vi "TEST SCREEN UPDATE_2.vi"(0 "Station in 1":refnum<class "Modbus Master.lvclass">, 3 "Staion  in error 2":errorcluster, 5 "Staion  in error 3":errorcluster, 6 "DataBase connection in":T11, 7 "Database error in":errorcluster, 21 "Staion  in error 1":errorcluster) -> (1 "Staion Error Out 1":errorcluster, 20 "Staion Out 1":refnum<k5>, 22 "Staion Out 2":refnum<k5>, 23 "Staion Error Out 2":errorcluster, 24 "Staion Out 3":refnum<k5>, 25 "Staion Error Out 3":errorcluster, 26 "Database connection out":T11, 27 "Database error out":errorcluster)   [LabVIEW 2024]
uses:
  <vilib>/addons/database/Connection.llb/Conn ObjectReference.ctl
  Controls/OP10_Cluster.ctl
  Controls/OP20_Cluster.ctl
  Controls/OP30_Cluster.ctl
  Controls/OP30_1_Cluster.ctl
  Controls/OP40_1_Cluster.ctl
  Controls/OP40_Cluster.ctl
  Controls/OP40_2_Cluster.ctl
  Controls/OP40_3_Cluster.ctl
  <vilib>/NI/Modbus Library/API/Master/Modbus Master.lvclass
  Controls/Data_Cluster_1.ctl
  test sequnece leak.ctl
  test setting.ctl
  Data base/database cluster.ctl
  Variable/Global.vi
  <vilib>/NI/Modbus Library/API/Wrapper/Create TCP Master.vi
  Support/Message Queue/Message Queue.lvlib
  <vilib>/NI/Modbus Library/API/Wrapper/API Main.lvlib
  <vilib>/addons/database/NI_Database_API.lvlib
panel:
  out "Staion Out 3":refnum<class "Modbus Master.lvclass">
  out "Staion Out 2":refnum<class "Modbus Master.lvclass">
  in  "Staion  in 3":refnum<class "Modbus Master.lvclass">
  in  "Station in 2":refnum<class "Modbus Master.lvclass">
  out "Staion Out 1":refnum<class "Modbus Master.lvclass">
  out "Communication error 3":bool
  out "Communication error 2":bool
  out "Communication error 1":bool
  in  "Exit":bool
  in  "Tab Control":enum32{"Screen_1", "Screen_2", "Other"}(tab)
  out "OP_30_1":T1
  out "OP_30":T2
  out "OP_20":T3
  out "OP_10":T4
  out "Result":string[][](table)
  out "OP_40_3":T5
  out "OP_40_2":T6
  out "OP_40":T7
  out "OP_40_1":T8
  in  "Tab Control 2":T9(tab)
  out "OP_10":string[](array[string])=["L095 1 28100M75T20-5PK 021224 A 0016", "ng", "OK", "OK", "OK", "OK"]
  in  "M 1":T10
  out "OP_10":u16[][](array[numeric])
  out "OP_10":sgl[][](array[numeric])
  in  "M 2":T10
  out "OP_20":string[](array[string])=["L095 1 28100M75T20-5PK 021224 A 2222", "KO", "KO", "KO", "K0"]
  out "OP_20":u16[][](array[numeric])
  out "OP_20":sgl[][](array[numeric])
  in  "M 3":T10
  out "OP_30":string[](array[string])
  out "OP_30":u16[][](array[numeric])
  out "OP_30":sgl[][](array[numeric])=[[0.0], [0.0], [0.0], [0.0], [0.0], [0.0], [0.0], [0.0], [1322.2], [485.2], [1271.9677], [0.0]]
  in  "M 4":T10
  in  "Barcode Already 4":bool
  in  "Barcode NG 4":bool
  in  "Barcode OK 4":bool
  out "OP_40":string[](array[string])
  out "OP_40":sgl[][](array[numeric])=[[0.0], [0.0], [0.0], [0.0], [1.38], [88.84], [0.0], [11.91], [16.25], [0.0], [0.0], [0.0], [0.0], [-30.7], [30.7], [0.0], [0.0], [-21.4], [26.7], [4.4], [21.91], [6.25], [0.0], [0.0], [0.0], [0.0]]
  out "OP_40":u16[][](array[numeric])=[[0], [0], [0], [0], [0], [0], [0], [0], [0], [0], [0], [0], [0], [0], [0], [52429], [52429], [0], [0], [0], [0], [0], [0], [0], [0], [0]]
  out "OP_10_CHLD":sgl[][](array[numeric])
  out "OP_10_CHLD 3":u16[][](array[numeric])=[[0], [175], [0], [0], [84], [0], [0], [585], [0], [0], [160], [0]]
  out "OP_10_CHLD 2":string[](array[string])=["12020499 234188 040324 500111       ", "", "5001", "11\u0000\u0000        12000089 0808/24  191124", "", "5023", "12000192 240073 050424 500111       ", "", "5001", "1200", "", "1202"]
  out "OP_20_CHLD 2":sgl[][](array[numeric])
  out "OP_20_CHLD 3":u16[][](array[numeric])=[[0], [722], [0], [0], [86], [0], [0], [86], [0]]
  out "OP_20_CHLD":string[](array[string])
  out "OP_30_CHLD":u16[][](array[numeric])=[[0], [175], [0]]
  out "OP_30_CHLD":string[](array[string])=["12020499 234188 040324 500111       ", "", "120204"]
  out "OP_30_CHLD":sgl[][](array[numeric])
  out "OP_40_CHLD 2":string[](array[string])
  out "OP_40_CHLD 3":u16[][](array[numeric])
  out "OP_40_CHLD":sgl[][](array[numeric])
  out "sr. out BARCODE":i32
  out "sr. out Laser":i32
  out "length":i32
  out "CommLoopCount":i32
  out "CommLoopCount 2":i32
  out "CommLoopCount 3":i32
  out "path for Laser sr":path
  out "path for Barcode sr.":path
  in  "Model NAME":string
  in  "count Path":path=path "D:/Configuration Folder Barcode/srno"
  in  "Visible":bool
  out "Exit 3":bool
  in  "TEST SETTING PATH":path=path "D:/Data Actuator/config/Settings"
  in  "Setting":path=path "D:/data/Test Settings"
  # "Test Screen"
  # "TESTING DATALOGGING SYSTEM"
  # "Station  OP 10"
  # "Station  OP 20"
  # "Station  OP 30"
  # "Station  OP 30_1"
  # "Station  OP 40"
  # "Station  OP 40_1"
  # "Station  OP 40_2"
  # "Station  OP 40_3"
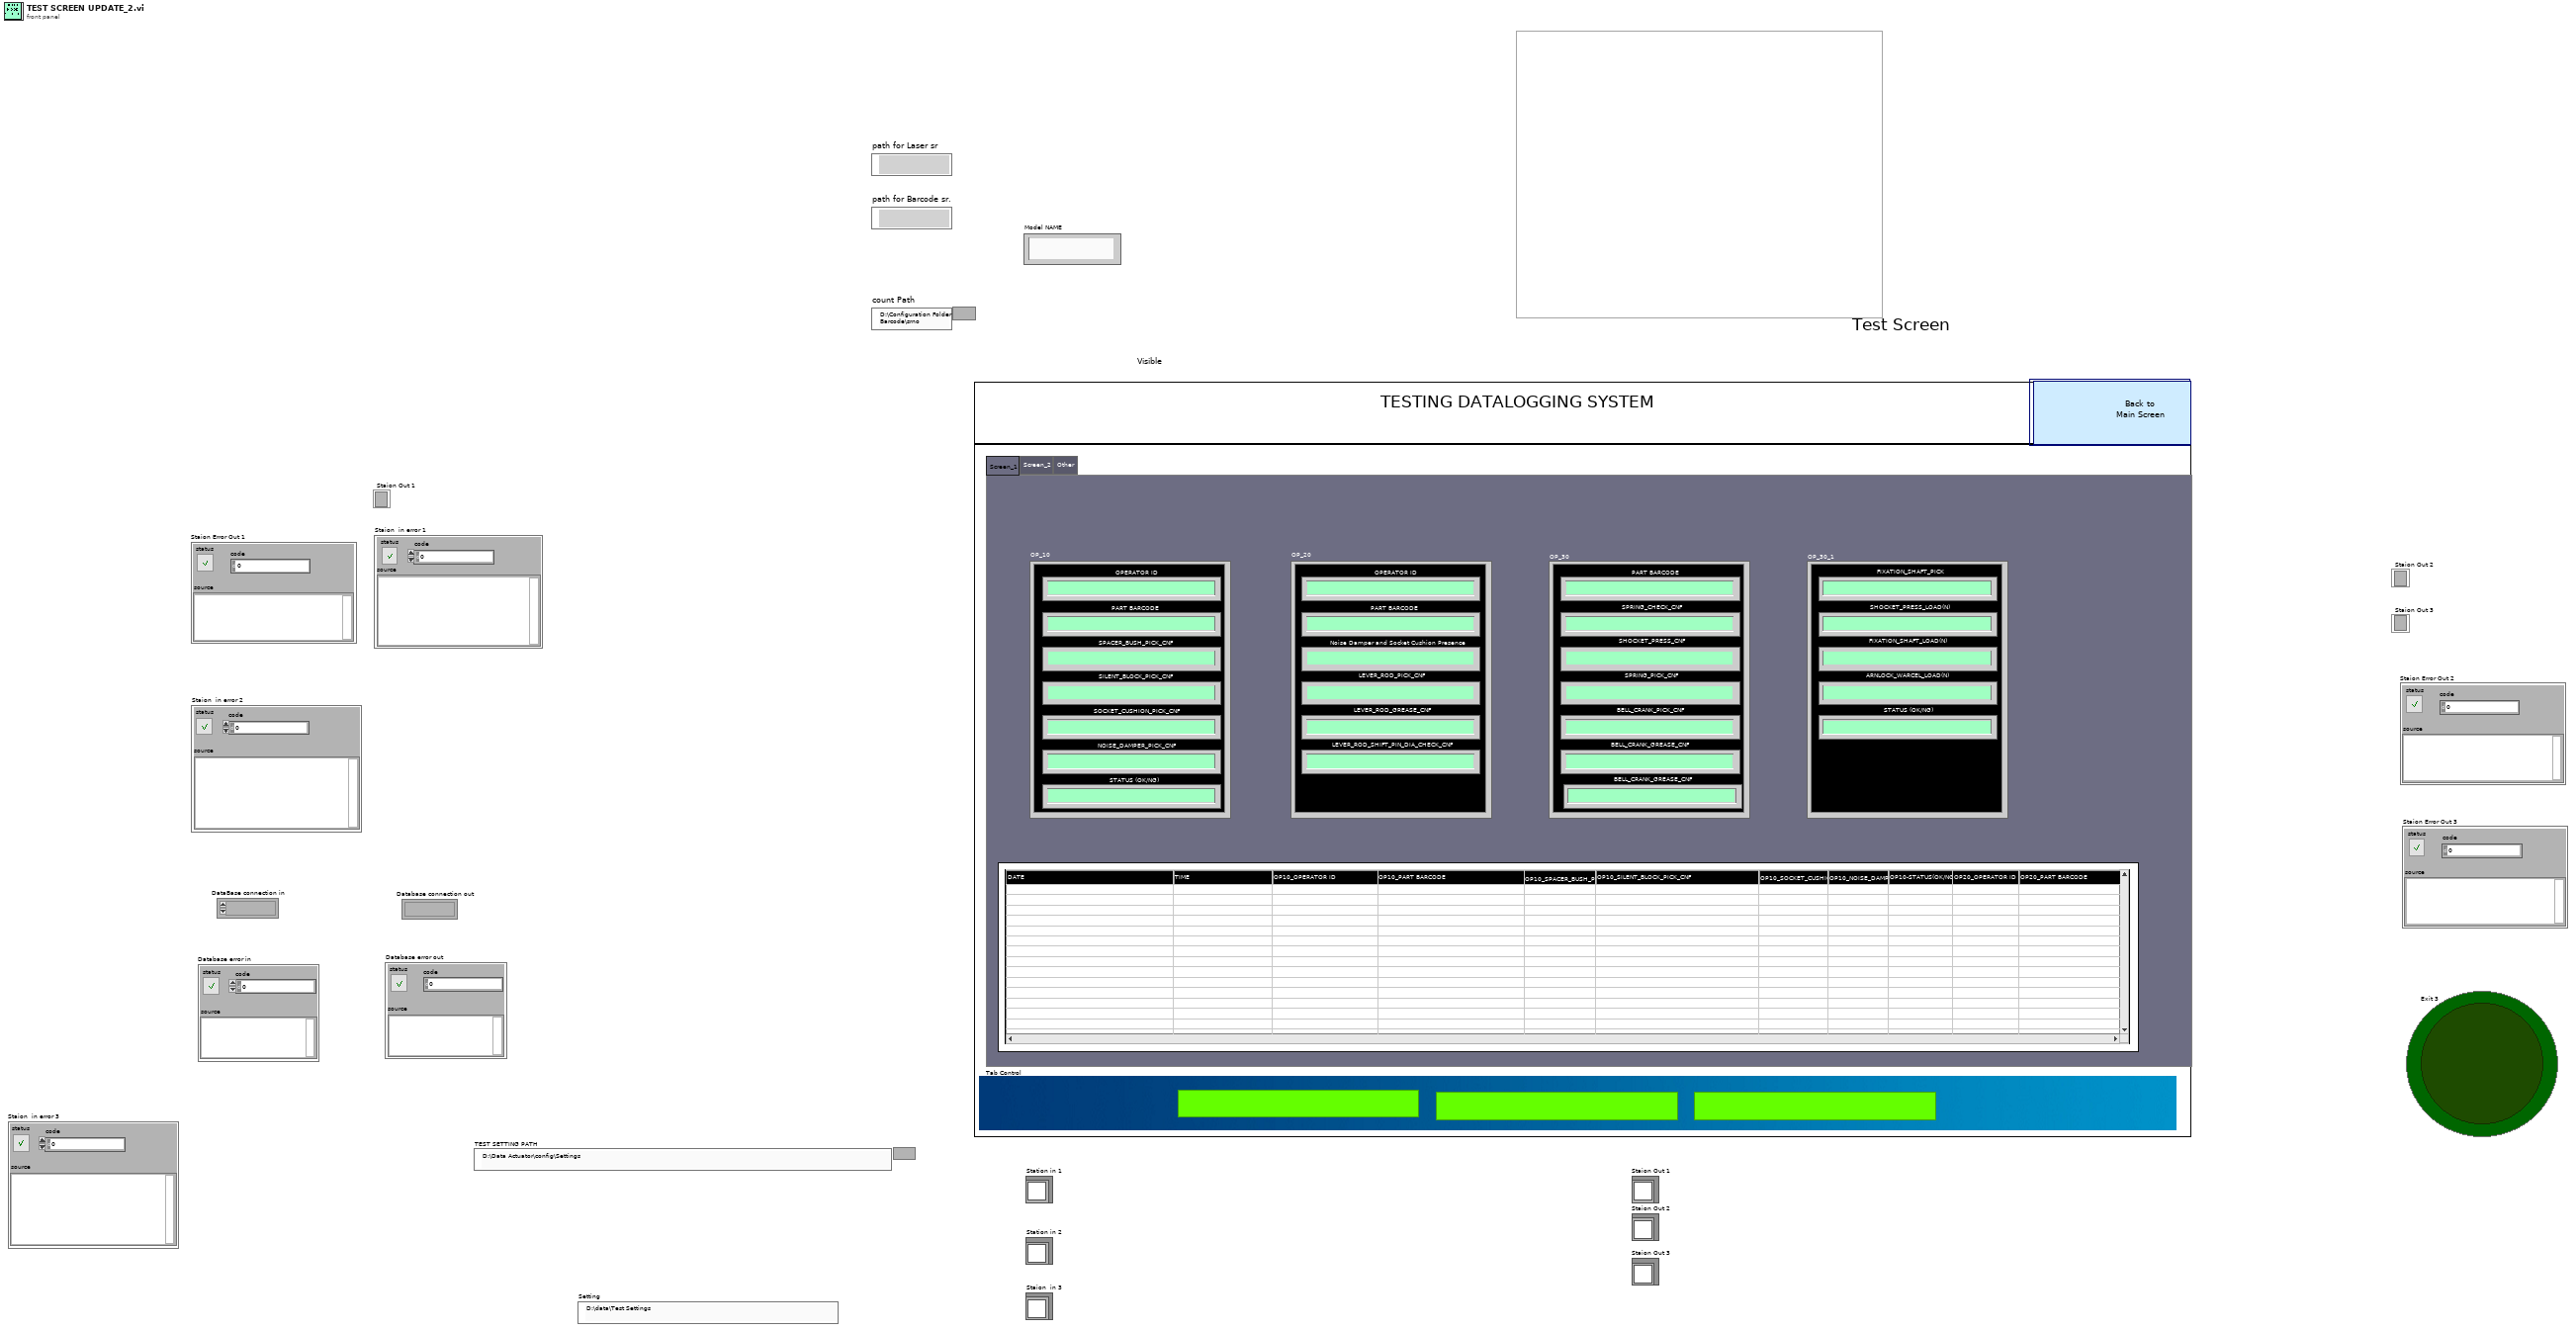
[diagram p1: front panel]
types:
  T1 = typedef "OP30_1_Cluster.ctl" = cluster{"FIXATION_SHAFT_PICK   ":string, "SHOCKET_PRESS_LOAD(N) ":string, "FIXATION_SHAFT_LOAD(N)":string, "ARNLOCK_WARCEL_LOAD(N)":string, "STATUS (OK/NG)":string}
  T2 = typedef "OP30_Cluster.ctl" = cluster{"PART BARCODE  ":string, "SPRING_CHECK_CNF ":string, "SHOCKET_PRESS_CNF":string, "SPRING_PICK_CNF":string, "BELL_CRANK_PICK_CNF":string, "BELL_CRANK_GREASE_CNF":string, "BELL_CRANK_GREASE_CNF":string}
  T3 = typedef "OP20_Cluster.ctl" = cluster{"OPERATOR ID ":string, "PART BARCODE ":string, "Noise Damper and Socket Cushion Presence":string, "LEVER_ROD_PICK_CNF":string, "LEVER_ROD_GREASE_CNF":string, "LEVER_ROD_SHIFT_PIN_DIA_CHECK_CNF":string}
  T4 = typedef "OP10_Cluster.ctl" = cluster{"OPERATOR ID ":string, "PART BARCODE ":string, "SPACER_BUSH_PICK_CNF":string, "SILENT_BLOCK_PICK_CNF":string, "SOCKET_CUSHION_PICK_CNF":string, "NOISE_DAMPER_PICK_CNF":string, "STATUS (OK/NG)":string}
  T5 = typedef "OP40_3_Cluster.ctl" = cluster{"SELECT_1ST_2ND_LOAD(N)":string, "SELECT_5TH_REV_LOAD(N) ":string, "HYSTERISIS CONFIRMATION":string, "PUNCH CONFIRMATION":string, "PDI FIXTURE CONFIRMATION":string, "EOL OK BARCODE SCAN CNF":string, "STATUS (OK/NG)":string}
  T6 = typedef "OP40_2_Cluster.ctl" = cluster{"PART BARCODE ":string, "SHIFT_2ND_4TH_REV_TRAVEL ":string, "SHIFT_1ST_3RD_5TH_TRAVEL ":string, "SHIFT_2ND_4TH_REV_LOAD(N)":string, "SHIFT_1ST_3RD_5TH_LOAD(N)":string, "SELECT_1ST_2ND_TRAVEL":string, "SELECT_5TH_REV_TRAVEL":string}
  T7 = typedef "OP40_Cluster.ctl" = cluster{"OPERATOR ID ":string, "PART BARCODE ":string, "BOOT_ORIENTATION_CHECK_CNF":string, "3_BOND_CONFIRMATION":string, "STATUS (OK/NG)":string, "PRETIGHT ANGLE":string, "POST TIGHT ANGLE":string}
  T8 = typedef "OP40_1_Cluster.ctl" = cluster{"KNOB TIGHT BARCODE OK ":string, "MAX KNOB TORQUE ":string, "NO. OF TURNS":string, "HEIGHT CHECK":string, "2 MM GAUGE CHECK":string, "STATUS (OK/NG)":string, "OPERATOR ID":string}
  T9 = enum32{"OP_10", "OP_20", "OP_30", "OP_40", "OP_10_CHILD", "OP_20_CHILD", "OP_30_CHILD", "OP_40_CHILD"}
  T10 = cluster{"Test Start Leak":bool, "Test Stop Leak":bool, "Scan Barcode":bool, "Test Running":bool, "Test OK":bool, "Test NG":bool, "Spare 1":bool, "Spare 2":bool}
  T11 = typedef "NI_Database_API.lvlib/Conn ObjectReference.ctl" = refnum<k1>
  T12 = typedef "Data_Cluster_1.ctl" = cluster{"OP_10":T4, "OP_20":T3, "OP_30":T2, "OP_30_1":T1, "OP_40":T7, "OP_40_1":T8, "OP_40_2":T6, "OP_40_3":T5}
  T13 = enum16{"open", "replace", "create", "open or create", "replace or create", "replace or create with confirmation"}
  T14 = typedef "test setting.ctl" = cluster{"M&M Part No.":string, "Vendor Code":string, "Part Identification Code":string, "Next Barcode Printing Wait Time":i32, "Path for LAser":path}
  T15 = typedef "test sequnece leak.ctl" = enum16{"Intilize", "CYCLE RESET", "Wait For teststart", "wait for scan", "check Barcode", "wait for start", "Wait for result", "wait for complete", "test stop", "Wait for LAser Scan Data", "check Scan Laser Data", "data save", "update tabel", "send data to Laser", "wait for Laser Start", "wait for laser stop"}
  T16 = typedef "database cluster.ctl" = cluster{"ID":i64, "Datetime":string, "PARTBARCODE":string, "TORQUE":string, "RESULT1":string, "CHILD1":string, "CHILD2":string, "CHILD3":string, "CHILD4":string, "RESULT2":string, "FINALBARCODE":string, "RESULT3":string, "REMARK":string, "OTHER":string}
  T17 = typedef "Communication setting.ctl" = cluster{"Light Scanner Port":refnum<visa-resource-name>, "Shift-A":timestamp, "Shift-B":timestamp, "Shift-C":timestamp, "Leak Scanner Port":refnum<visa-resource-name>, "Barcode Printer":refnum<visa-resource-name>}
  T18 = cluster{"[0]":string, "[1]":string, "[2]":string, "[3]":string, "[4]":string, "[5]":string, "[6]":string}
  T19 = cluster{"[0]":string, "[1]":string, "[2]":string, "[3]":string, "[4]":string, "[5]":string}
  T20 = cluster{"[0]":string, "[1]":string, "[2]":string, "[3]":string, "[4]":string}
  T21 = cluster{"OP_30[0]":string, "OP_30[1]":string, "OP_30[2]":string, "OP_30[3]":string, "OP_30[4]":string, "OP_30[5]":string, "OP_30[6]":string}
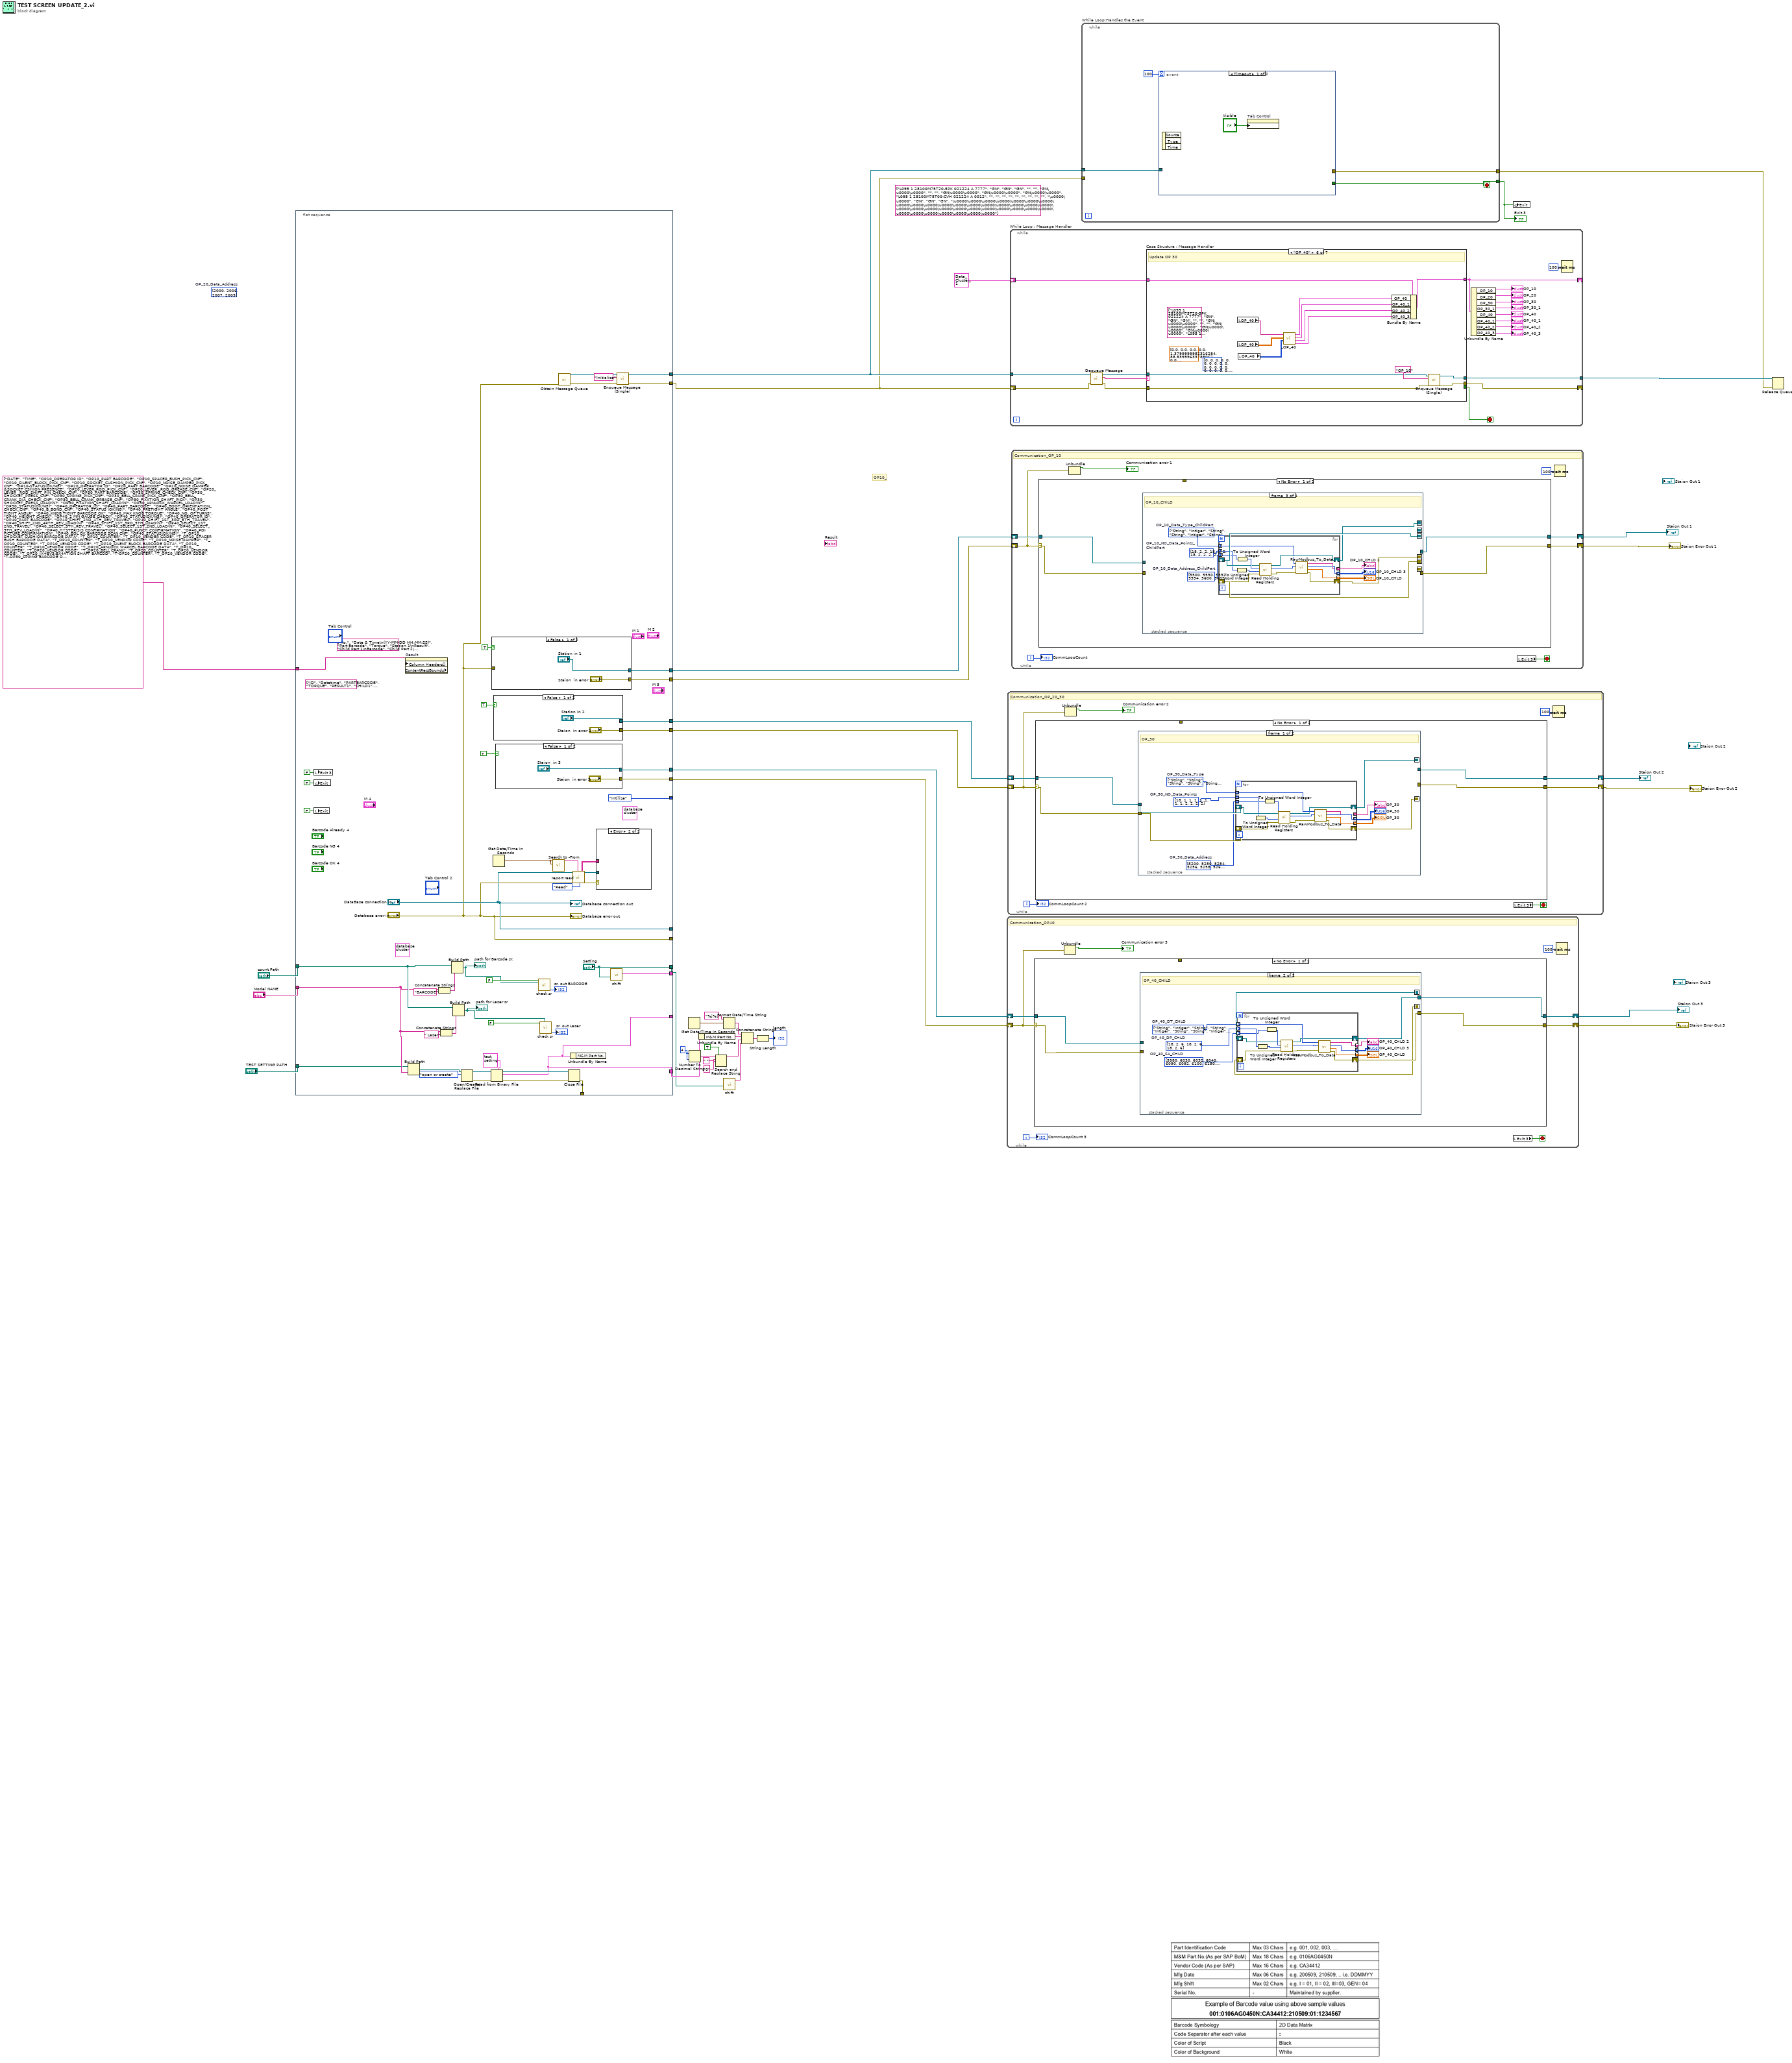
[diagram p0: block diagram]
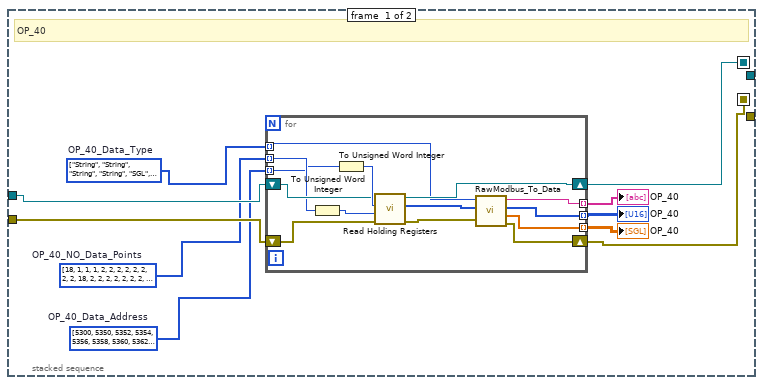
[diagram p2: hidden frame]
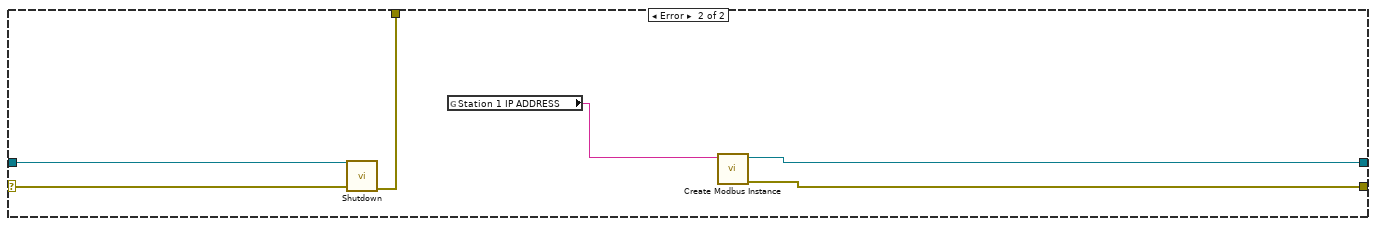
[diagram p3: hidden frame]
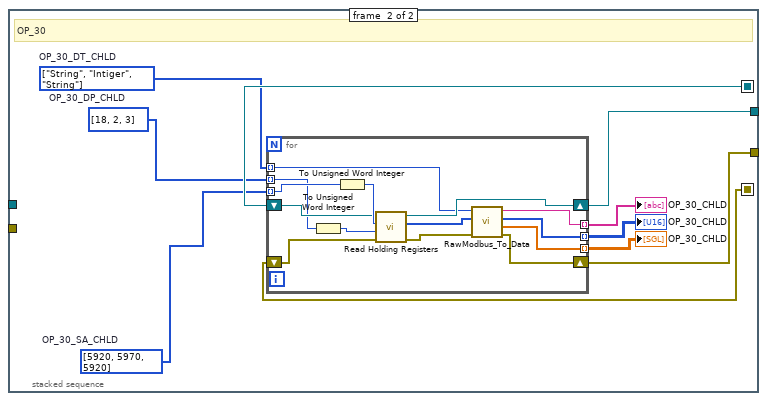
[diagram p4: hidden frame]
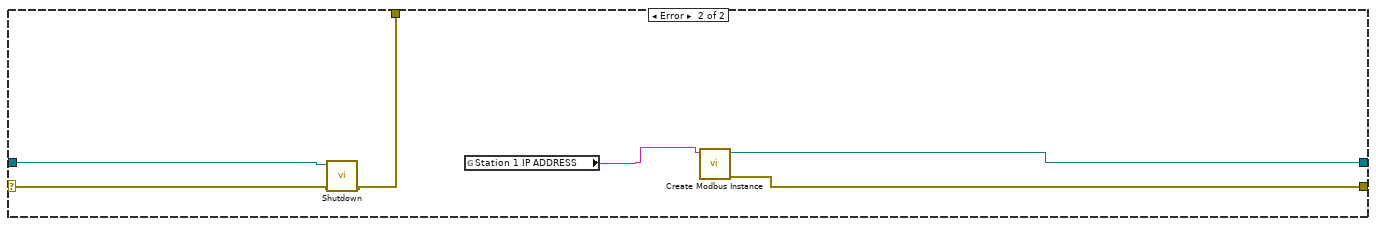
[diagram p5: hidden frame]
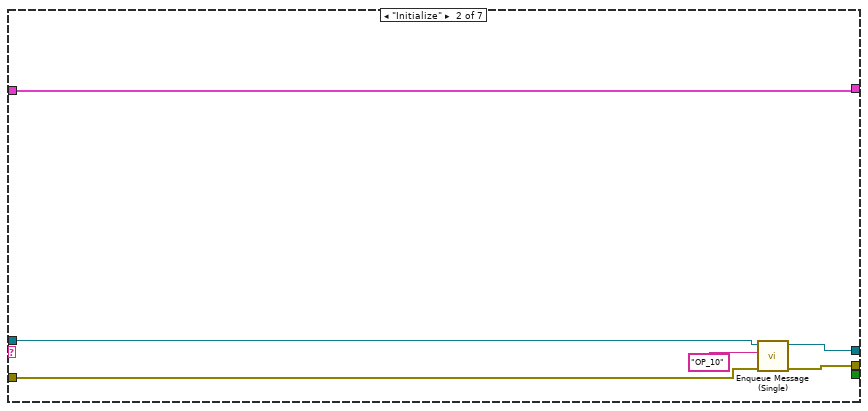
[diagram p7: hidden frame]
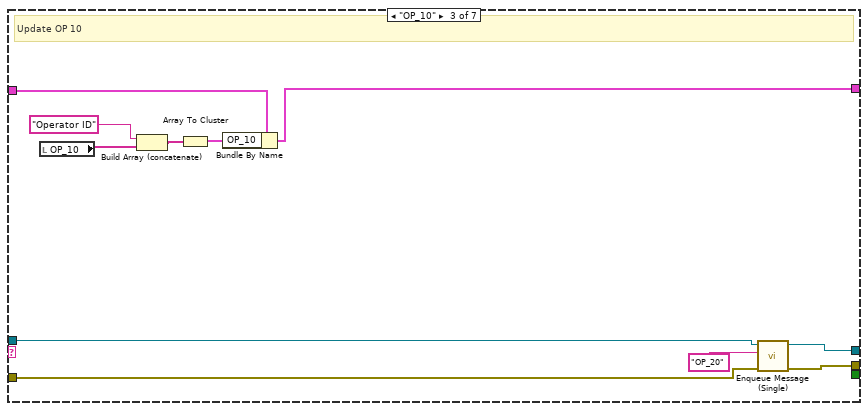
[diagram p8: hidden frame]
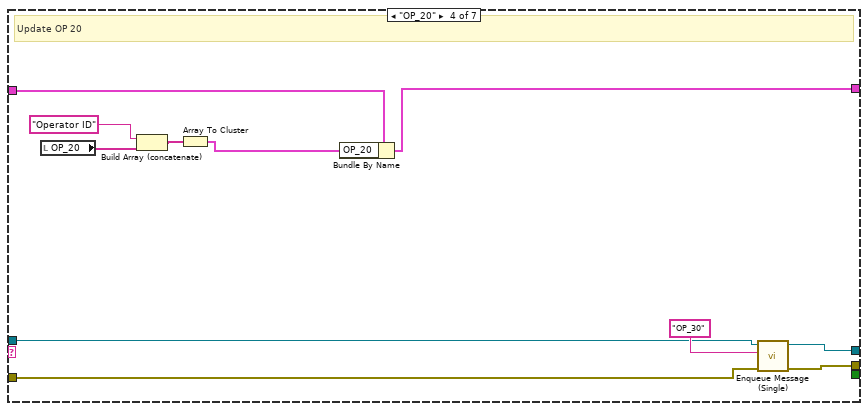
[diagram p9: hidden frame]
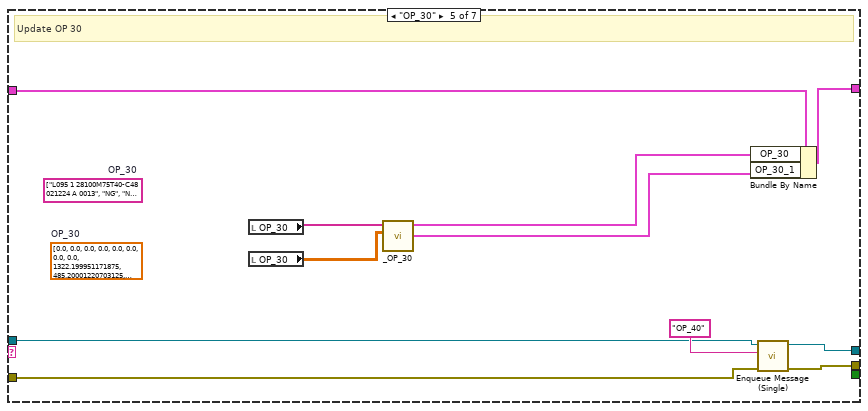
[diagram p10: hidden frame]
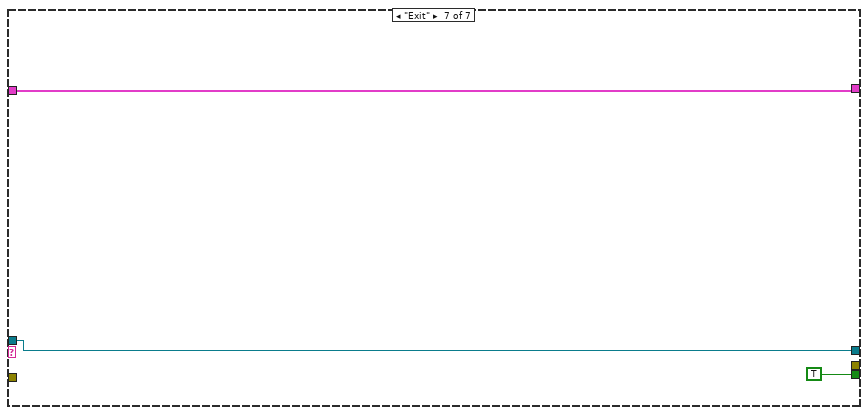
[diagram p11: hidden frame]
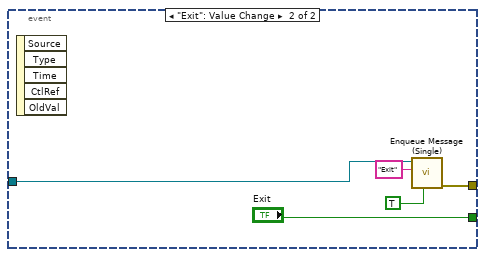
[diagram p12: hidden frame]
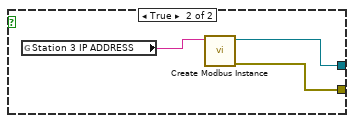
[diagram p13: hidden frame]
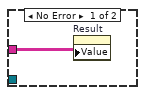
[diagram p14: hidden frame]
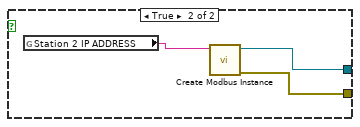
[diagram p15: hidden frame]
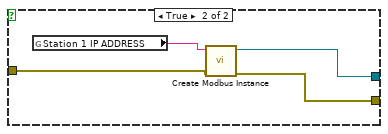
[diagram p16: hidden frame]
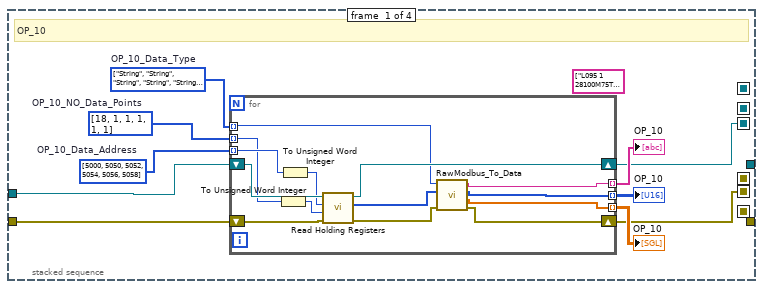
[diagram p17: hidden frame]
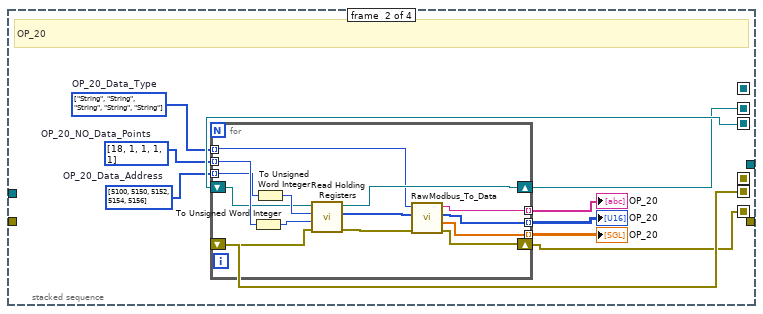
[diagram p18: hidden frame]
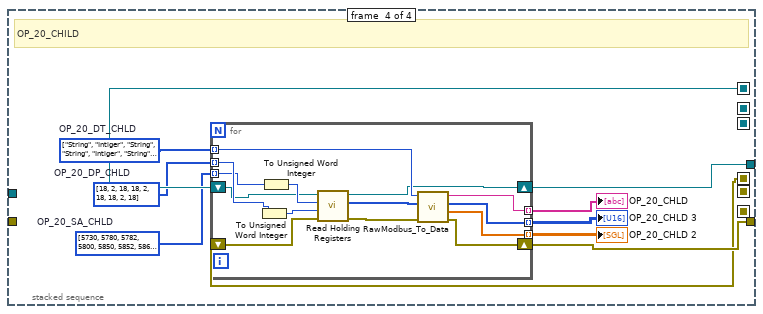
[diagram p19: hidden frame]
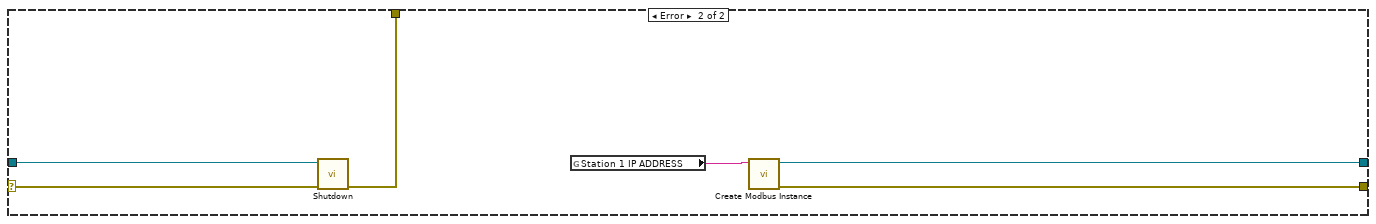
[diagram p20: hidden frame]
diagram:
  (unwired) string[] ["L095 1 28100M75T20-5PK 021224 A 7777", "GN", "GN", "GN", "", "", "GN\u0000\u0000", "", "", "GN\u0000\u0000", "GN\u0000\u0000", "GN\u0000\u0000", "L095 1 28100M75T00-CVH 021224 A 0012", "", "", "", "", "", "", "", "", "", "\u0000\u0000", "GN", "GN", "GN", "\u0000\u0000\u0000\u0000\u0000\u0000\u0000\u0000\u0000\u0000\u0000\u0000\u0000\u0000\u0000\u0000\u0000\u0000\u0000\u0000\u0000\u0000\u0000\u0000\u0000\u0000\u0000\u0000\u0000\u0000\u0000\u0000\u0000\u0000\u0000\u0000"] ("OP_40")
  (unwired) i32[] [2000, 2006, 2007, 2009]  # OP_20_Data_Address
  w20 = i16 4 ("width (-)")
  # "OP10_"
  n1 = flat-sequence {
    tunnel: ["Setting"] -> w19
    tunnel: [w87] -> _
    tunnel: [w85] -> w36
    tunnel: [w84] -> w35
    tunnel: [test_sequnece_leak."Intilize" ("Enum 2")] -> _
    tunnel: [w78] -> w10
    tunnel: [w77] -> w9
    tunnel: ["DataBase connection in"] -> _
    tunnel: ["Database error in"] -> _
    tunnel: [w64] -> _
    tunnel: [w49] -> _
    tunnel: "count Path" -> [w52]
    tunnel: "Model NAME" -> [w51]
    tunnel: "TEST SETTING PATH" -> [w50]
    tunnel: [w49] -> w21
    tunnel: [w47] -> w8
    tunnel: [w46] -> w7
    tunnel: string[] ["DATE", "TIME", "OP10_OPERATOR ID", "OP10_PART BARCODE", "OP10_SPACER_BUSH_PICK_CNF", "OP10_SILENT_BLOCK_PICK_CNF", "OP10_SOCKET_CUSHION_PICK_CNF", "OP10_NOISE_DAMPER_PICK_CNF", "OP10-STATUS(OK/NG)", "OP20_OPERATOR ID", "OP20_PART BARCODE", "OP20_NOISE DAMPER &SOCKET CSHION PRESENCE", "OP20_LEVER_ROD_PICK_CNF", "OP20_LEVER _ROD_GREASE_CNF", "OP20_LEVER _ROD_SHIFT_PIN_CHECK_CNF", "OP30_PART BARCODE", "OP30_SPRING_CHECK_CNF", "OP30_SHOCKET_PRESS_CNF", "OP30_SPRING_PICK_CNF", "OP30_BELL_CRANK_PICK_CNF", "OP30_BELL_CRANK_DIA_CHECK_CNF", "OP30_BELL_CRANK_GREASE_CNF", "OP30_FIXATION_SHAFT_PICK", "OP30_SHOCKET_PRESS_LOAD(N)", "OP30_FIXATION_SHAFT_LOAD(N)", "OP30_ARNLOCK_WARCEL_LOAD(N)", "OP30_STATUS(OK/NG)", "OP40_OPERATOR_ID", "OP40_PART_BARCODE", "OP40_BOOT_ORIENTATION_CHECK_CNF", "OP40_B_BOND_CNF", "OP40_STATUS (OK/NG)", "OP40_PRETIGHT ANGLE", "OP40_POST TIGHT ANGLR", "OP40_KNOB TIGHT BARCODE OK", "OP40_MAX KNOB TORQUE", "OP40_NO. OF TURNS", "OP40_HEIGHT CHECK", "OP40_2 MM GAUGE CHECK", "OP40_STATUS(OK/NG)", "OP40_OPERATOR ID", "OP40_PART BARCODE", "OP40_SHIFT_2ND_4TH_REV_TRAVEL", "OP40_SHIFT_1ST_3RD_5TH_TRAVEL", "OP40_SHIFT_2ND_4RTH_REV_LOAD(N)", "OP40_SHIFT_1ST_3RD_5TH_LOAD(N)", "OP40_SELECT_1ST_2ND_TRAVEL", "OP40_SELECT_5TH_REV_TRAVEL", "OP40_SELECT_1ST_2ND_LOAD(N)", "OP40_SELECT_5TH_REV_LOAD(N)", "OP40_HYSTERISIS CONFIRMATION", "OP40_PUNCH CONFIRMATION", "OP40_PDI FICTURE CONFIRMATION", "OP40_EOL OK BARCODE SCAN CNF", "OP40_STATUS(OK/NG)", "T_OP10_SHOCKET CUSHION BARCODE DATA", "T_OP10_COUNTER", "T_OP10_VENDER CODE", "T_OP10_SPACER BUSH BARCODE DATA", "T_OP10_COUNTER", "T_OP10_VENDOR CODE", "T_OP10_NOISE DAMPER", "T_OP10_COUNTER", "T_OP10_VENDOR CODE", "T_OP10_SILENT BLOCK BARCODE DATA", "T_OP10_COUNTER", "T_OP10_VENDOR CODE", "T_OP20_ARNLOCK WARCEL BARCODE DATA", "T_OP20_COUNTER", "T_OP20_VENDOR CODE", "T_OP20_BELL CRANK", "T_OP20_COUNTER", "T_OP20_VENDOR CODE", "T_OP20_IX+BV3:BX4ATION SHAFT BARCOD", "T-OP20_COUNTER", "T_OP20_VENDOR CODE", "T-OP30_SPRING BARCODE DAT", "T-OP30_COUNTER", "T_OP30_VENDOR CODE", "T_OP40_KNOB BARCODE DAT", "T_OP40_COUNTER", "T_OP40_VENDOR CODE", "T_OP40_DELUX BARCODE DATA", "T-OP40_COUNTER", "T_OP40_VENDOR CODE", "T_OP40_INSERT LOCK BARCODE DATA", "T_OP40_COUNTER", "T_OP40_VENDOR CODE"] ("appended array") -> [w45]
    tunnel: [w42] -> w14
    tunnel: [w40] -> w15
    frame #0 {
      (unwired) string[] ["ID", "Datetime", "PARTBARCODE", "TORQUE", "RESULT1", "CHILD1", "CHILD2", "CHILD3", "CHILD4", "RESULT2", "FINALBARCODE", "RESULT3", "REMARK", "OTHER"] ("tables")
      (unwired) T16 {"ID"=0, "Datetime"="", "PARTBARCODE"="", "TORQUE"="", "RESULT1"="", "CHILD1"="", "CHILD2"="", "CHILD3"="", "CHILD4"="", "RESULT2"="", "FINALBARCODE"="", "RESULT3"="", "REMARK"="", "OTHER"=""} ("Data")
      (unwired) string[] ["No.", "Date & Time\n(YY-MM-DD HH:MM:SS)", "Part Barcode", "Torque", "Station 1\nResult", "Child Part 1\nBarcode", "Child Part 2\nBarcode", "Child Part 3\nBarcode", "Child Part 4\nBarcode", "Station 2\nResult", "Final Part\nBarcode", "Remark", "Other"] ("Column Header Strings[]")
      (unwired) T16 {"ID"=0, "Datetime"="", "PARTBARCODE"="", "TORQUE"="", "RESULT1"="", "CHILD1"="", "CHILD2"="", "CHILD3"="", "CHILD4"="", "RESULT2"="", "FINALBARCODE"="", "RESULT3"="", "REMARK"="", "OTHER"=""} ("Data")
      n2 = local write "Exit 3"(FALSE ("Exit 3")) -> ()
      n3 = global write "Global.vi" "Exit"(FALSE ("Exit")) -> ()
      n4 = local write "Exit"(FALSE ("Exit")) -> ()
      n5 = property on="Result" class="Tbl (strict)" props=["Column Headers[]", "ContentRectBounds"]("Column Headers[]"=w45) -> ()  [unwired: 2 in, 3 out]
      n6 = Build Path(base path=w50, name or relative path=w51) -> (appended path=w66:path)
      n7 = Concatenate Strings(w51, "BARCODE" ("string")) -> (w72:string)
      n8 = Concatenate Strings(w51, " Laser" ("string")) -> (w57:string)
      n9 = Build Path(base path=w52, name or relative path=w72) -> (appended path=w73:path)
      "path for Barcode sr." <- w73
      n10 = Build Path(base path=w52, name or relative path=w57) -> (appended path=w56:path)
      "path for Laser sr" <- w56
      n11 = Open/Create/Replace File(file path (use dialog)=w66, operation (0:open)=T13."open or create") -> (refnum out=w71:refnum<file>, error out=w70:errorcluster)  [unwired: 4 in, 1 out]
      n12 = Read from Binary File(5:T14 {"M&M Part No."="", "Vendor Code"="02BHMSI1009190338RKWPG", "Part Identification Code"="02CRMTT1009190250KWPG", "Next Barcode Printing Wait Time"=0, "Path for LAser"=path ""} ("Cluster"), 8:w70, 11:w71) -> (0:w69:errorcluster, 2:w49:T14, 3:w68:refnum<file>)  [unwired: 3 in, 1 out]
      n13 = case shown="False" TRUE {
        tunnel: ["Station in 1" w102] -> w85
        tunnel: ["Staion  in error 1" w103] -> w84
        tunnel: "Database error in" -> [_ w104]
        frame False {
        }
        frame True {
          n14 = global read "Global.vi" "Station 1 IP ADDRESS"() -> (w105:string)
          n15 = call-poly <vilib>:"Create Modbus Instance.vi"("error in"=w104, "address"=w105) -> ("error out"=w103:errorcluster, "TCP master instance"=w102:refnum<class "Modbus Master.lvclass">)  [unwired: 8 in]
        }
      }
      n16 = Get Date/Time In Seconds() -> (seconds since 1Jan1904=w63:timestamp)
      n17 = case shown="False" TRUE {
        tunnel: ["Station in 2" w98] -> w78
        tunnel: ["Staion  in error 2" w97] -> w77
        frame False {
        }
        frame True {
          n18 = global read "Global.vi" "Station 2 IP ADDRESS"() -> (w99:string)
          n19 = call-poly <vilib>:"Create Modbus Instance.vi"("address"=w99) -> ("error out"=w97:errorcluster, "TCP master instance"=w98:refnum<class "Modbus Master.lvclass">)  [unwired: 9 in]
        }
      }
      n20 = case shown="False" TRUE {
        tunnel: ["Staion  in 3" w91] -> w47
        tunnel: ["Staion  in error 3" w92] -> w46
        frame False {
        }
        frame True {
          n21 = global read "Global.vi" "Station 3 IP ADDRESS"() -> (w93:string)
          n22 = call-poly <vilib>:"Create Modbus Instance.vi"("address"=w93) -> ("error out"=w92:errorcluster, "TCP master instance"=w91:refnum<class "Modbus Master.lvclass">)  [unwired: 9 in]
        }
      }
      n23 = call "check sr.vi"("file path (use dialog)"=w73, "writeL:t"=FALSE) -> ("sr. out"=→"sr. out BARCODE":i32)  [unwired: 9 in]
      n24 = call "check sr.vi"("file path (use dialog)"=w56, "writeL:t"=FALSE) -> ("sr. out"=→"sr. out Laser":i32)  [unwired: 9 in]
      n25 = call "Search to -From.vi"("From date"=w63, "To Date"=w63) -> ("search dataString"=w61:string)  [unwired: 9 in]
      n26 = call "Obtain Message Queue.vi"("error in (no error)"="Database error in") -> ("error out"=w43:errorcluster, "Message Queue"=w41:refnum<queue>)  [unwired: 9 in]
      n27 = Close File(refnum=w68, error in=w69) -> (error out=w64:errorcluster)  [unwired: 1 out]
      n28 = Unbundle By Name(w49) -> ()  [unwired: 1 out]
      n29 = call "report read.vi"("connection reference"="DataBase connection in", "error in (no error)"="Database error in", "search dataString"=w61, "Enum"=enum16{"Write", "Read"}."Read") -> ("Search Reverse"=w60:string[][], "connection reference out"=w59:T11, "error out"=w44:errorcluster)  [unwired: 10 in, 3 out]
      n30 = case shown="Error" w44 {
        tunnel: w60 -> [w94 _]
        tunnel: w59 -> [_ _]
        frame No Error {
          n31 = property on="Result" class="Tbl (strict)"("Value"=w94) -> ()  [unwired: 2 in, 2 out]
        }
        frame Error {
        }
      }
      n32 = call "shift.vi"("Setting"="Setting") -> ("data"=w87:T17)  [unwired: 9 in, 1 out]
      n33 = call "Enqueue Message (Single).vi"("error in (no error)"=w43, "Message"="Initialize", "Message Queue"=w41) -> ("error out"=w42:errorcluster, "dup Message Queue"=w40:refnum<queue>)  [unwired: 7 in]
      "Database connection out" <- "DataBase connection in"
      "Database error out" <- "Database error in"
    }
  }
  n34 = Get Date/Time In Seconds() -> (seconds since 1Jan1904=w26:timestamp)
  n35 = Number To Decimal String(number=w20, width (-)=w20) -> (decimal integer string=w22:string)
  n36 = Unbundle By Name(w21) -> ("M&M Part No."=w30:string)
  n37 = Search and Replace String(replace all?=TRUE ("replace all? (F)"), input string=w22, search string=" ", replace string="0" ("replace string (\"\")")) -> (result string=w25:string)  [unwired: 4 in, 3 out]
  n38 = Format Date/Time String(time format string (%c)="%j%y", seconds (now)=w26) -> (date/time string=w29:string)  [unwired: 1 in]
  n39 = call "shift.vi"("Setting"=w19) -> ("SHIFT_A"=w18:string)  [unwired: 9 in, 1 out]
  n40 = Concatenate Strings(w29, w30, w25, w18) -> (w17:string)
  n41 = String Length(string=w17) -> (length=→"length":i32)
  n42 = while {
    shift-right: [w113] -> w2
    shift-left: w8 -> [w112]
    shift-right: [w111] -> w5
    shift-left: w7 -> [w110]
    i -> [w107]
    stop <- w109 stop-if-true
    # "Communication_OP40"
    n43 = case shown="No Error" w110 {
      selector: w110 -> [w116 w166]
      tunnel: [w114 w171] -> w113
      tunnel: [w115 w170] -> w111
      tunnel: w112 -> [w117 w167]
      tunnel: [_ w168] -> _
      frame No Error {
        n44 = stacked-sequence {
          seq-local: [w119 _] -> [_ w149]
          seq-local: [w118 _] -> [_ w148]
          tunnel: [_ w151] -> w114
          tunnel: [_ w150] -> w115
          tunnel: w117 -> [w124 _]
          tunnel: w116 -> [w123 _]
          frame #0 {
            w120 = i32[] [5300, 5350, 5352, 5354, 5356, 5358, 5360, 5362, 5364, 5366, 5368, 5370, 5400, 5450, 5452, 5456, 5458, 5460, 5462, 5464, 5466, 5468, 6570, 5472, 5474, 5476, 5300]  # OP_40_Data_Address
            w121 = i32[] [18, 1, 1, 1, 2, 2, 2, 2, 2, 2, 2, 2, 18, 2, 2, 2, 2, 2, 2, 2, 2, 2, 1, 1, 1, 1, 2]  # OP_40_NO_Data_Points
            w122 = enum16{"String", "Intiger", "DBL", "SGL"}[] [enum."String", enum."String", enum."String", enum."String", enum."SGL", enum."SGL", enum."String", enum."SGL", enum."SGL", enum."String", enum."String", enum."String", enum."String", enum."SGL", enum."SGL", enum."Intiger", enum."Intiger", enum."SGL", enum."SGL", enum."SGL", enum."SGL", enum."SGL", enum."String", enum."String", enum."String", enum."String"] items=["String", "Intiger", "DBL", "SGL"]  # OP_40_Data_Type
            # "OP_40"
            n45 = for {
              tunnel: [w137] -> w127 mode=indexing
              shift-right: [w133] -> w119
              shift-left: w124 -> [w130]
              shift-right: [w134] -> w118
              shift-left: w123 -> [w131]
              tunnel: w120 -> [w128] mode=indexing
              tunnel: w121 -> [w129] mode=indexing
              tunnel: [w135] -> w125 mode=indexing
              tunnel: [w136] -> w126 mode=indexing
              tunnel: w122 -> [w132] mode=indexing
              n46 = To Unsigned Word Integer(number=w129) -> (unsigned 16bit integer=w140:u16)
              n47 = To Unsigned Word Integer(number=w128) -> (unsigned 16bit integer=w141:u16)
              n48 = call-dynamic "Read Holding Registers.vi"("error in"=w131, "number of inputs"=w140, "starting address"=w141, "Modbus master in"=w130) -> ("error out"=w138:errorcluster, "register values"=w139:u16[], "Modbus master out"=w133:refnum<class "Modbus Master.lvclass">)  [unwired: 5 in]
              n49 = call "RawModbus_To_Data.vi"("ErrorIn"=w138, "InpuData"=w139, "Read Data Type"=w132) -> ("ErrorOut"=w134:errorcluster, "Array"=w135:sgl[], "16bit integer"=w136:i16[], "String"=w137:string)  [unwired: 5 in]
            }
            "OP_40" <- w127
            "OP_40" <- w126
            "OP_40" <- w125
          }
          frame #1 {
            w147 = i32[] [5980, 6030, 6032, 6040, 6090, 6092, 6100, 6150, 6152]  # OP_40_SA_CHLD
            w145 = i32[] [18, 2, 6, 18, 2, 6, 18, 2, 6]  # OP_40_DP_CHLD
            w146 = enum16{"String", "Intiger", "DBL", "SGL"}[] [enum."String", enum."Intiger", enum."String", enum."String", enum."Intiger", enum."String", enum."String", enum."Intiger", enum."String"] items=["String", "Intiger", "DBL", "SGL"]  # OP_40_DT_CHLD
            # "OP_40_CHILD"
            n50 = for {
              tunnel: [w154] -> w144 mode=indexing
              shift-right: [w155] -> w151
              shift-left: w149 -> [w157]
              shift-right: [w161] -> w150
              shift-left: w148 -> [w160]
              tunnel: w147 -> [w158] mode=indexing
              tunnel: w145 -> [w159] mode=indexing
              tunnel: [w152] -> w142 mode=indexing
              tunnel: [w153] -> w143 mode=indexing
              tunnel: w146 -> [w156] mode=indexing
              n51 = To Unsigned Word Integer(number=w159) -> (unsigned 16bit integer=w164:u16)
              n52 = To Unsigned Word Integer(number=w158) -> (unsigned 16bit integer=w165:u16)
              n53 = call-dynamic "Read Holding Registers.vi"("error in"=w160, "number of inputs"=w164, "starting address"=w165, "Modbus master in"=w157) -> ("error out"=w162:errorcluster, "register values"=w163:u16[], "Modbus master out"=w155:refnum<class "Modbus Master.lvclass">)  [unwired: 5 in]
              n54 = call "RawModbus_To_Data.vi"("ErrorIn"=w162, "InpuData"=w163, "Read Data Type"=w156) -> ("ErrorOut"=w161:errorcluster, "Array"=w152:sgl[], "16bit integer"=w153:i16[], "String"=w154:string)  [unwired: 5 in]
            }
            "OP_40_CHLD 2" <- w144
            "OP_40_CHLD 3" <- w143
            "OP_40_CHLD" <- w142
          }
        }
      }
      frame Error {
        n55 = call-dynamic "Shutdown.vi"("error in"=w166, "Modbus master in"=w167) -> ("error out"=w168:errorcluster)  [unwired: 9 in]
        n56 = global read "Global.vi" "Station 1 IP ADDRESS"() -> (w169:string)
        n57 = call-poly <vilib>:"Create Modbus Instance.vi"("address"=w169) -> ("error out"=w170:errorcluster, "TCP master instance"=w171:refnum<class "Modbus Master.lvclass">)  [unwired: 9 in]
      }
    }
    n58 = Unbundle(w110) -> ("status"=→"Communication error 3":bool)  [unwired: 2 out]
    n59 = local read "Exit 3"() -> (w109:bool)
    n60 = Wait (ms)(milliseconds to wait=u32 100) -> ()  [unwired: 1 out]
    "CommLoopCount 3" <- w107
  }
  "Staion Error Out 3" <- w5
  "Staion Out 3" <- w2
  n61 = while {
    shift-right: [w179] -> w3
    shift-left: w10 -> [w178]
    shift-right: [w177] -> w6
    shift-left: w9 -> [w176]
    i -> [w173]
    stop <- w175 stop-if-true
    # "Communication_OP_20_30"
    n62 = case shown="No Error" w176 {
      selector: w176 -> [w180 w234]
      tunnel: [w183 w232] -> w179
      tunnel: [w182 w237] -> w177
      tunnel: w178 -> [w181 w233]
      tunnel: [_ w235] -> _
      frame No Error {
        n63 = stacked-sequence {
          seq-local: [w187 _] -> [_ w212]
          seq-local: [w186 _] -> [_ w211]
          tunnel: w180 -> [w189 _]
          tunnel: w181 -> [w188 _]
          tunnel: [_ w217] -> w183
          tunnel: [_ w216] -> w182
          frame #0 {
            w193 = enum16{"String", "Intiger", "DBL", "SGL"}[] [enum."String", enum."String", enum."String", enum."String", enum."String", enum."String", enum."String", enum."String", enum."SGL", enum."SGL", enum."SGL", enum."String"] items=["String", "Intiger", "DBL", "SGL"]  # OP_30_Data_Type
            w184 = i32[] [18, 1, 1, 1, 1, 1, 1, 1, 2, 2, 2, 2]  # OP_30_NO_Data_Points
            w185 = i32[] [5200, 5250, 5254, 5256, 5258, 5260, 5262, 5100, 5266, 5268, 5270, 5272]  # OP_30_Data_Address
            # "OP_30"
            n64 = for {
              tunnel: [w199] -> w192 mode=indexing
              shift-right: [w197] -> w187
              shift-left: w188 -> [w196]
              shift-right: [w203] -> w186
              shift-left: w189 -> [w202]
              tunnel: w185 -> [w194] mode=indexing
              tunnel: w184 -> [w195] mode=indexing
              tunnel: [w201] -> w190 mode=indexing
              tunnel: [w200] -> w191 mode=indexing
              tunnel: w193 -> [w198] mode=indexing
              n65 = To Unsigned Word Integer(number=w195) -> (unsigned 16bit integer=w206:u16)
              n66 = To Unsigned Word Integer(number=w194) -> (unsigned 16bit integer=w207:u16)
              n67 = call-dynamic "Read Holding Registers.vi"("error in"=w202, "number of inputs"=w206, "starting address"=w207, "Modbus master in"=w196) -> ("error out"=w204:errorcluster, "register values"=w205:u16[], "Modbus master out"=w197:refnum<class "Modbus Master.lvclass">)  [unwired: 5 in]
              n68 = call "RawModbus_To_Data.vi"("ErrorIn"=w204, "InpuData"=w205, "Read Data Type"=w198) -> ("ErrorOut"=w203:errorcluster, "Array"=w201:sgl[], "16bit integer"=w200:i16[], "String"=w199:string)  [unwired: 5 in]
            }
            "OP_30" <- w192
            "OP_30" <- w191
            "OP_30" <- w190
          }
          frame #1 {
            w209 = i32[] [5920, 5970, 5920]  # OP_30_SA_CHLD
            w208 = i32[] [18, 2, 3]  # OP_30_DP_CHLD
            w210 = enum16{"String", "Intiger", "DBL", "SGL"}[] [enum."String", enum."Intiger", enum."String"] items=["String", "Intiger", "DBL", "SGL"]  # OP_30_DT_CHLD
            # "OP_30"
            n69 = for {
              tunnel: [w227] -> w215 mode=indexing
              shift-right: [w223] -> w217
              shift-left: w212 -> [w221]
              shift-right: [w224] -> w216
              shift-left: w211 -> [w220]
              tunnel: w209 -> [w219] mode=indexing
              tunnel: w208 -> [w218] mode=indexing
              tunnel: [w225] -> w213 mode=indexing
              tunnel: [w226] -> w214 mode=indexing
              tunnel: w210 -> [w222] mode=indexing
              n70 = To Unsigned Word Integer(number=w218) -> (unsigned 16bit integer=w230:u16)
              n71 = To Unsigned Word Integer(number=w219) -> (unsigned 16bit integer=w231:u16)
              n72 = call-dynamic "Read Holding Registers.vi"("error in"=w220, "number of inputs"=w230, "starting address"=w231, "Modbus master in"=w221) -> ("error out"=w228:errorcluster, "register values"=w229:u16[], "Modbus master out"=w223:refnum<class "Modbus Master.lvclass">)  [unwired: 5 in]
              n73 = call "RawModbus_To_Data.vi"("ErrorIn"=w228, "InpuData"=w229, "Read Data Type"=w222) -> ("ErrorOut"=w224:errorcluster, "Array"=w225:sgl[], "16bit integer"=w226:i16[], "String"=w227:string)  [unwired: 5 in]
            }
            "OP_30_CHLD" <- w215
            "OP_30_CHLD" <- w214
            "OP_30_CHLD" <- w213
          }
        }
      }
      frame Error {
        n74 = call-dynamic "Shutdown.vi"("error in"=w234, "Modbus master in"=w233) -> ("error out"=w235:errorcluster)  [unwired: 9 in]
        n75 = global read "Global.vi" "Station 1 IP ADDRESS"() -> (w236:string)
        n76 = call-poly <vilib>:"Create Modbus Instance.vi"("address"=w236) -> ("error out"=w237:errorcluster, "TCP master instance"=w232:refnum<class "Modbus Master.lvclass">)  [unwired: 9 in]
      }
    }
    n77 = Unbundle(w176) -> ("status"=→"Communication error 2":bool)  [unwired: 2 out]
    n78 = local read "Exit 3"() -> (w175:bool)
    n79 = Wait (ms)(milliseconds to wait=u32 100) -> ()  [unwired: 1 out]
    "CommLoopCount 2" <- w173
  }
  "Staion Error Out 2" <- w6
  "Staion Out 2" <- w3
  n80 = while "While Loop : Message Handler" {
    tunnel: w15 -> [w255]
    tunnel: [w250] -> w13
    shift-right: [w248] -> _
    shift-left: w14 -> [w256]
    shift-right: [w246] -> _
    shift-left: T12 {"OP_10"={"OPERATOR ID "="", "PART BARCODE "="", "SPACER_BUSH_PICK_CNF"="", "SILENT_BLOCK_PICK_CNF"="", "SOCKET_CUSHION_PICK_CNF"="", "NOISE_DAMPER_PICK_CNF"="", "STATUS (OK/NG)"=""}, "OP_20"={"OPERATOR ID "="", "PART BARCODE "="", "Noise Damper and Socket Cushion Presence"="", "LEVER_ROD_PICK_CNF"="", "LEVER_ROD_GREASE_CNF"="", "LEVER_ROD_SHIFT_PIN_DIA_CHECK_CNF"=""}, "OP_30"={"PART BARCODE  "="", "SPRING_CHECK_CNF "="", "SHOCKET_PRESS_CNF"="", "SPRING_PICK_CNF"="", "BELL_CRANK_PICK_CNF"="", "BELL_CRANK_GREASE_CNF"="", "BELL_CRANK_GREASE_CNF"=""}, "OP_30_1"={"FIXATION_SHAFT_PICK   "="", "SHOCKET_PRESS_LOAD(N) "="", "FIXATION_SHAFT_LOAD(N)"="", "ARNLOCK_WARCEL_LOAD(N)"="", "STATUS (OK/NG)"=""}, "OP_40"={"OPERATOR ID "="", "PART BARCODE "="", "BOOT_ORIENTATION_CHECK_CNF"="", "3_BOND_CONFIRMATION"="", "STATUS (OK/NG)"="", "PRETIGHT ANGLE"="", "POST TIGHT ANGLE"=""}, "OP_40_1"={"KNOB TIGHT BARCODE OK "="", "MAX KNOB TORQUE "="", "NO. OF TURNS"="", "HEIGHT CHECK"="", "2 MM GAUGE CHECK"="", "STATUS (OK/NG)"="", "OPERATOR ID"=""}, "OP_40_2"={"PART BARCODE "="", "SHIFT_2ND_4TH_REV_TRAVEL "="", "SHIFT_1ST_3RD_5TH_TRAVEL "="", "SHIFT_2ND_4TH_REV_LOAD(N)"="", "SHIFT_1ST_3RD_5TH_LOAD(N)"="", "SELECT_1ST_2ND_TRAVEL"="", "SELECT_5TH_REV_TRAVEL"=""}, "OP_40_3"={"SELECT_1ST_2ND_LOAD(N)"="", "SELECT_5TH_REV_LOAD(N) "="", "HYSTERISIS CONFIRMATION"="", "PUNCH CONFIRMATION"="", "PDI FIXTURE CONFIRMATION"="", "EOL OK BARCODE SCAN CNF"="", "STATUS (OK/NG)"=""}} ("Data Cluster") -> [w247]
    stop <- w251 stop-if-true
    n81 = call "Dequeue Message.vi"("error in (no error)"=w256, "Message Queue"=w255) -> ("error out"=w254:errorcluster, "Message"=w253:string, "dup Message Queue"=w252:refnum<queue>)  [unwired: 6 in, 1 out]
    n82 = case "Case Structure : Message Handler" shown="\"OP_40\"" w253 {
      tunnel: w254 -> [_ w264 w275 w286 w297 w311 _]
      tunnel: w252 -> [w258 w261 w272 w283 w294 w308 w313]
      tunnel: [_ _ _ _ _ _ TRUE] -> w251
      tunnel: [w258 w260 w271 w282 w293 w307 w313] -> w250
      tunnel: [_ w263 w274 w285 w296 w310 _] -> w248
      tunnel: w247 -> [w257 w259 w266 w279 w292 w306 w312]
      tunnel: [w257 w259 w265 w278 w291 w305 w312] -> w246
      frame "False", Default {
      }
      frame "Initialize" {
        n83 = call "Enqueue Message (Single).vi"("error in (no error)"=w264, "Message"="OP_10", "Message Queue"=w261) -> ("error out"=w263:errorcluster, "dup Message Queue"=w260:refnum<queue>)  [unwired: 7 in]
      }
      frame "OP_10" {
        # "Update OP 10"
        n84 = local read "OP_10"() -> (w270:string[])
        n85 = Build Array (concatenate)("Operator ID", w270) -> (w268:string[])
        n86 = Array To Cluster(array=w268) -> (cluster=w267:T18)
        n87 = Bundle By Name(cluster=w266, "OP_10"=w267) -> (w265:T12)
        n88 = call "Enqueue Message (Single).vi"("error in (no error)"=w275, "Message"="OP_20", "Message Queue"=w272) -> ("error out"=w274:errorcluster, "dup Message Queue"=w271:refnum<queue>)  [unwired: 7 in]
      }
      frame "OP_20" {
        # "Update OP 20"
        n89 = local read "OP_20"() -> (w277:string[])
        n90 = Build Array (concatenate)("Operator ID", w277) -> (w280:string[])
        n91 = Array To Cluster(array=w280) -> (cluster=w276:T19)
        n92 = Bundle By Name(cluster=w279, "OP_20"=w276) -> (w278:T12)
        n93 = call "Enqueue Message (Single).vi"("error in (no error)"=w286, "Message"="OP_30", "Message Queue"=w283) -> ("error out"=w285:errorcluster, "dup Message Queue"=w282:refnum<queue>)  [unwired: 7 in]
      }
      frame "OP_30" {
        (unwired) sgl[][] [[0.0], [0.0], [0.0], [0.0], [0.0], [0.0], [0.0], [0.0], [1322.2], [485.2], [1265.9], [0.0]]  # OP_30
        (unwired) string[] ["L095 1 28100M75T40-C48 021224 A 0013", "NG", "NG", "NG", "NG", "NG", "NG", "NG", "", "", "", "NG\u0000\u0000"]  # OP_30
        # "Update OP 30"
        n94 = local read "OP_30"() -> (w288:string[])
        n95 = local read "OP_30"() -> (w287:sgl[][])
        n96 = call "_OP_30.vi"("OP_30 3"=w287, "OP_30 in"=w288) -> ("Cluster"=w290:T20, "OP_30 out"=w289:T21)  [unwired: 8 in]
        n97 = Bundle By Name(cluster=w292, "OP_30"=w289, "OP_30_1"=w290) -> (w291:T12)
        n98 = call "Enqueue Message (Single).vi"("error in (no error)"=w297, "Message"="OP_40", "Message Queue"=w294) -> ("error out"=w296:errorcluster, "dup Message Queue"=w293:refnum<queue>)  [unwired: 7 in]
      }
      frame "OP_40" {
        (unwired) u16[][] [[0, 0], [0, 0], [0, 0], [0, 0], [0, 0], [0, 0], [0, 0], [0, 0], [0, 0], [0, 0], [0, 0], [0, 0], [0, 0], [0, 0], [0, 0], [52429, 16268], [52429, 16268], [0, 0], [0, 0], [0, 0], [0, 0], [0, 0], [0, 0], [0, 0], [0, 0], [0, 0], [0, 0]] ("OP_40")
        (unwired) sgl[][] [[0.0], [0.0], [0.0], [0.0], [1.38], [88.84], [0.0], [11.91], [16.25], [0.0], [0.0], [0.0], [0.0], [-30.7], [30.7], [0.0], [0.0], [-21.4], [26.7], [4.4], [21.91], [6.25], [0.0], [0.0], [0.0], [0.0], [0.0]] ("OP_40")
        (unwired) string[] ["L095 1 28100M75T20-5PK 021224 A 7777", "GN", "GN", "GN", "", "", "GN\u0000\u0000", "", "", "GN\u0000\u0000", "GN\u0000\u0000", "GN\u0000\u0000", "L095 1 28100M75T00-CVH 021224 A 0012", "", "", "", "", "", "", "", "", "", "\u0000\u0000", "GN", "GN", "GN", "\u0000\u0000\u0000\u0000\u0000\u0000\u0000\u0000\u0000\u0000\u0000\u0000\u0000\u0000\u0000\u0000\u0000\u0000\u0000\u0000\u0000\u0000\u0000\u0000\u0000\u0000\u0000\u0000\u0000\u0000\u0000\u0000\u0000\u0000\u0000\u0000"] ("OP_40")
        # "Update OP 30"
        n99 = local read "OP_40"() -> (w298:string[])
        n100 = local read "OP_40"() -> (w300:sgl[][])
        n101 = local read "OP_40"() -> (w299:u16[][])
        n102 = call "_OP_40.vi"("OP_40_Integer"=w299, "OP_40_Float"=w300, "OP_40_string"=w298) -> ("Cluster"=w301:T18, "Cluster 2"=w302:T18, "Cluster 3"=w303:T18, "Cluster 4"=w304:T18)  [unwired: 5 in]
        n103 = Bundle By Name(cluster=w306, "OP_40"=w304, "OP_40_1"=w303, "OP_40_2"=w302, "OP_40_3"=w301) -> (w305:T12)
        n104 = call "Enqueue Message (Single).vi"("error in (no error)"=w311, "Message"="OP_10", "Message Queue"=w308) -> ("error out"=w310:errorcluster, "dup Message Queue"=w307:refnum<queue>)  [unwired: 7 in]
      }
      frame "Exit" {
      }
    }
    n105 = Unbundle By Name(w246) -> ("OP_10"=→"OP_10":T4, "OP_20"=→"OP_20":T3, "OP_30"=→"OP_30":T2, "OP_30_1"=→"OP_30_1":T1, "OP_40"=→"OP_40":T7, "OP_40_1"=→"OP_40_1":T8, "OP_40_2"=→"OP_40_2":T6, "OP_40_3"=→"OP_40_3":T5)
    n106 = Wait (ms)(milliseconds to wait=u32 100) -> ()  [unwired: 1 out]
  }
  n107 = while {
    shift-right: [w322] -> w4
    shift-left: w36 -> [w321]
    shift-right: [w320] -> w37
    shift-left: w35 -> [w319]
    i -> [w316]
    stop <- w318 stop-if-true
    # "Communication_OP_10"
    n108 = case shown="No Error" w319 {
      selector: w319 -> [w325 w427]
      tunnel: [w324 w424] -> w322
      tunnel: [w323 w428] -> w320
      tunnel: w321 -> [w326 w423]
      tunnel: [_ w426] -> _
      frame No Error {
        n109 = stacked-sequence {
          seq-local: [w327 _ _ _] -> [_ w360 w384 _]
          seq-local: [w328 _ _ _] -> [_ w359 w383 _]
          seq-local: [_ w358 _ _] -> [_ _ _ _]
          seq-local: [_ w357 _ _] -> [_ _ _ _]
          seq-local: [_ _ w381 _] -> [_ _ _ w405]
          seq-local: [_ _ w382 _] -> [_ _ _ w406]
          tunnel: [_ _ _ w407] -> w324
          tunnel: [_ _ _ w408] -> w323
          tunnel: w326 -> [w336 _ _ _]
          tunnel: w325 -> [w335 _ _ _]
          frame #0 {
            (unwired) string[] ["L095 1 28100M75T20-5PK 021224 A 0016", "OK", "OK", "OK", "OK", "OK"] ("OP_10")
            w329 = i32[] [5000, 5050, 5052, 5054, 5056, 5058]  # OP_10_Data_Address
            w330 = i32[] [18, 1, 1, 1, 1, 1]  # OP_10_NO_Data_Points
            w331 = enum16{"String", "Intiger", "DBL", "SGL"}[] [enum."String", enum."String", enum."String", enum."String", enum."String", enum."String"] items=["String", "Intiger", "DBL", "SGL"]  # OP_10_Data_Type
            # "OP_10"
            n110 = for {
              tunnel: [w341] -> w332 mode=indexing
              shift-right: [w344] -> w327
              shift-left: w336 -> [w349]
              shift-right: [w337] -> w328
              shift-left: w335 -> [w350]
              tunnel: w329 -> [w347] mode=indexing
              tunnel: w330 -> [w345] mode=indexing
              tunnel: [w343] -> w333 mode=indexing
              tunnel: [w342] -> w334 mode=indexing
              tunnel: w331 -> [w340] mode=indexing
              n111 = To Unsigned Word Integer(number=w345) -> (unsigned 16bit integer=w346:u16)
              n112 = To Unsigned Word Integer(number=w347) -> (unsigned 16bit integer=w348:u16)
              n113 = call-dynamic "Read Holding Registers.vi"("error in"=w350, "number of inputs"=w346, "starting address"=w348, "Modbus master in"=w349) -> ("error out"=w338:errorcluster, "register values"=w339:u16[], "Modbus master out"=w344:refnum<class "Modbus Master.lvclass">)  [unwired: 5 in]
              n114 = call "RawModbus_To_Data.vi"("ErrorIn"=w338, "InpuData"=w339, "Read Data Type"=w340) -> ("ErrorOut"=w337:errorcluster, "Array"=w343:sgl[], "16bit integer"=w342:i16[], "String"=w341:string)  [unwired: 5 in]
            }
            "OP_10" <- w332
            "OP_10" <- w334
            "OP_10" <- w333
          }
          frame #1 {
            w356 = enum16{"String", "Intiger", "DBL", "SGL"}[] [enum."String", enum."String", enum."String", enum."String", enum."String"] items=["String", "Intiger", "DBL", "SGL"]  # OP_20_Data_Type
            w355 = i32[] [18, 1, 1, 1, 1]  # OP_20_NO_Data_Points
            w354 = i32[] [5100, 5150, 5152, 5154, 5156]  # OP_20_Data_Address
            # "OP_20"
            n115 = for {
              tunnel: [w365] -> w353 mode=indexing
              shift-right: [w367] -> w358
              shift-left: w360 -> [w368]
              shift-right: [w371] -> w357
              shift-left: w359 -> [w362]
              tunnel: w354 -> [w369] mode=indexing
              tunnel: w355 -> [w370] mode=indexing
              tunnel: [w363] -> w351 mode=indexing
              tunnel: [w364] -> w352 mode=indexing
              tunnel: w356 -> [w366] mode=indexing
              n116 = To Unsigned Word Integer(number=w370) -> (unsigned 16bit integer=w373:u16)
              n117 = To Unsigned Word Integer(number=w369) -> (unsigned 16bit integer=w374:u16)
              n118 = call-dynamic "Read Holding Registers.vi"("error in"=w362, "number of inputs"=w373, "starting address"=w374, "Modbus master in"=w368) -> ("error out"=w361:errorcluster, "register values"=w372:u16[], "Modbus master out"=w367:refnum<class "Modbus Master.lvclass">)  [unwired: 5 in]
              n119 = call "RawModbus_To_Data.vi"("ErrorIn"=w361, "InpuData"=w372, "Read Data Type"=w366) -> ("ErrorOut"=w371:errorcluster, "Array"=w363:sgl[], "16bit integer"=w364:i16[], "String"=w365:string)  [unwired: 5 in]
            }
            "OP_20" <- w353
            "OP_20" <- w352
            "OP_20" <- w351
          }
          frame #2 {
            w376 = i32[] [5500, 5550, 5552, 5554, 5600, 5602, 5610, 5660, 5662, 5670, 5720, 5500]  # OP_10_Data_Address_ChildPart
            w375 = i32[] [18, 2, 2, 18, 2, 2, 18, 2, 2, 2, 2, 2]  # OP_10_NO_Data_Points_ChildPart
            w377 = enum16{"String", "Intiger", "DBL", "SGL"}[] [enum."String", enum."Intiger", enum."String", enum."String", enum."Intiger", enum."String", enum."String", enum."Intiger", enum."String", enum."String", enum."Intiger", enum."String"] items=["String", "Intiger", "DBL", "SGL"]  # OP_10_Data_Type_ChildPart
            # "OP_10_CHILD"
            n120 = for {
              tunnel: [w391] -> w380 mode=indexing
              shift-right: [w390] -> w381
              shift-left: w384 -> [w388]
              shift-right: [w394] -> w382
              shift-left: w383 -> [w389]
              tunnel: w376 -> [w386] mode=indexing
              tunnel: [w393] -> w378 mode=indexing
              tunnel: [w392] -> w379 mode=indexing
              tunnel: w377 -> [w385] mode=indexing
              tunnel: w375 -> [w387] mode=indexing
              n121 = To Unsigned Word Integer(number=w387) -> (unsigned 16bit integer=w397:u16)
              n122 = To Unsigned Word Integer(number=w386) -> (unsigned 16bit integer=w398:u16)
              n123 = call-dynamic "Read Holding Registers.vi"("error in"=w389, "number of inputs"=w397, "starting address"=w398, "Modbus master in"=w388) -> ("error out"=w395:errorcluster, "register values"=w396:u16[], "Modbus master out"=w390:refnum<class "Modbus Master.lvclass">)  [unwired: 5 in]
              n124 = call "RawModbus_To_Data.vi"("ErrorIn"=w395, "InpuData"=w396, "Read Data Type"=w385) -> ("ErrorOut"=w394:errorcluster, "Array"=w393:sgl[], "16bit integer"=w392:i16[], "String"=w391:string)  [unwired: 5 in]
            }
            "OP_10_CHLD 2" <- w380
            "OP_10_CHLD 3" <- w379
            "OP_10_CHLD" <- w378
          }
          frame #3 {
            w401 = i32[] [5730, 5780, 5782, 5800, 5850, 5852, 5860, 5910, 5730]  # OP_20_SA_CHLD
            w400 = i32[] [18, 2, 18, 18, 2, 18, 18, 2, 18]  # OP_20_DP_CHLD
            w399 = enum16{"String", "Intiger", "DBL", "SGL"}[] [enum."String", enum."Intiger", enum."String", enum."String", enum."Intiger", enum."String", enum."String", enum."Intiger", enum."String"] items=["String", "Intiger", "DBL", "SGL"]  # OP_20_DT_CHLD
            # "OP_20_CHILD"
            n125 = for {
              tunnel: [w418] -> w404 mode=indexing
              shift-right: [w409] -> w407
              shift-left: w405 -> [w411]
              shift-right: [w415] -> w408
              shift-left: w406 -> [w414]
              tunnel: w401 -> [w412] mode=indexing
              tunnel: [w416] -> w402 mode=indexing
              tunnel: [w417] -> w403 mode=indexing
              tunnel: w399 -> [w410] mode=indexing
              tunnel: w400 -> [w413] mode=indexing
              n126 = To Unsigned Word Integer(number=w413) -> (unsigned 16bit integer=w421:u16)
              n127 = To Unsigned Word Integer(number=w412) -> (unsigned 16bit integer=w422:u16)
              n128 = call-dynamic "Read Holding Registers.vi"("error in"=w414, "number of inputs"=w421, "starting address"=w422, "Modbus master in"=w411) -> ("error out"=w419:errorcluster, "register values"=w420:u16[], "Modbus master out"=w409:refnum<class "Modbus Master.lvclass">)  [unwired: 5 in]
              n129 = call "RawModbus_To_Data.vi"("ErrorIn"=w419, "InpuData"=w420, "Read Data Type"=w410) -> ("ErrorOut"=w415:errorcluster, "Array"=w416:sgl[], "16bit integer"=w417:i16[], "String"=w418:string)  [unwired: 5 in]
            }
            "OP_20_CHLD" <- w404
            "OP_20_CHLD 3" <- w403
            "OP_20_CHLD 2" <- w402
          }
        }
      }
      frame Error {
        n130 = call-dynamic "Shutdown.vi"("error in"=w427, "Modbus master in"=w423) -> ("error out"=w426:errorcluster)  [unwired: 9 in]
        n131 = global read "Global.vi" "Station 1 IP ADDRESS"() -> (w425:string)
        n132 = call-poly <vilib>:"Create Modbus Instance.vi"("address"=w425) -> ("error out"=w428:errorcluster, "TCP master instance"=w424:refnum<class "Modbus Master.lvclass">)  [unwired: 9 in]
      }
    }
    n133 = Unbundle(w319) -> ("status"=→"Communication error 1":bool)  [unwired: 2 out]
    n134 = local read "Exit 3"() -> (w318:bool)
    n135 = Wait (ms)(milliseconds to wait=u32 100) -> ()  [unwired: 1 out]
    "CommLoopCount" <- w316
  }
  "Staion Error Out 1" <- w37
  "Staion Out 1" <- w4
  n136 = while "While Loop:Handles the Event" {
    tunnel: [w431] -> w34
    tunnel: w15 -> [w430]
    tunnel: w14 -> [_]
    tunnel: [w429] -> w12
    stop <- w431 stop-if-true
    n137 = event shown="[0] Timeout" {
      selector: _ -> [_ _]
      dyn-events: _ -> [_ _]
      timeout: 100 -> [_ _]
      tunnel: [_ "Exit"] -> w431
      tunnel: w430 -> [_ w436]
      tunnel: [_ w434] -> w429
      event Timeout {
        n138 = event-data() -> ()  [unwired: 1 in, 3 out]
        n139 = property on="Tab Control" class="TabCtl (strict)"("Page Labels Display Visible?"="Visible") -> ()  [unwired: 2 in, 2 out]
      }
      event "Exit": Value Change {
        n140 = event-data() -> ()  [unwired: 1 in, 5 out]
        n141 = call "Enqueue Message (Single).vi"("Priority Message? (F)"=TRUE, "Message"="Exit", "Message Queue"=w436) -> ("error out"=w434:errorcluster)  [unwired: 7 in, 1 out]
      }
    }
  }
  "Exit 3" <- w34
  n142 = global write "Global.vi" "Exit"(w34) -> ()
  n143 = Release Queue(queue=w13, error in (no error)=w12) -> ()  [unwired: 1 in, 3 out]
